vi "Test ADC Rate.vi"() -> ()   [LabVIEW 2020, in "CTI-Visa-Scratchpad.lvlib"]
uses:
  CTI-Visa-Scratchpad.lvlib
  CTI-Visa/CTI-Visa.lvlib
  <vilib>/ptbypt/NI_PtbyPt.lvlib
panel:
  in  "stop":bool
  out "ADC":dbl[][](graph)=[[2063.0, 0.0007534999895142391, 756.5504025676244]]
  in  "Port":refnum<visa-resource-name>="COM3"
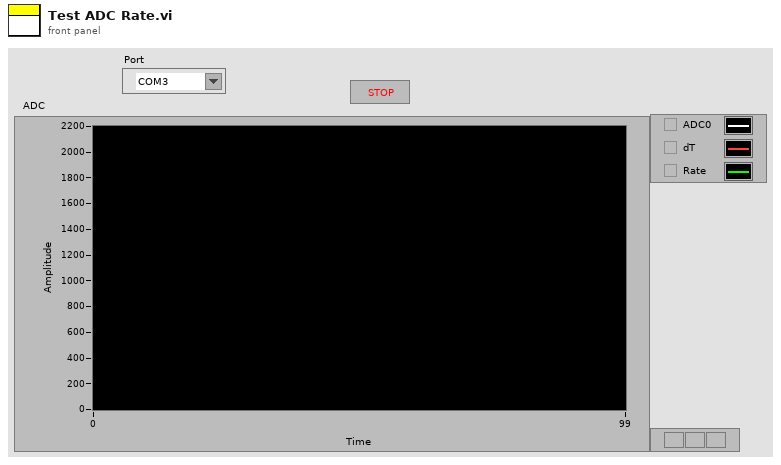
[diagram p1: front panel]
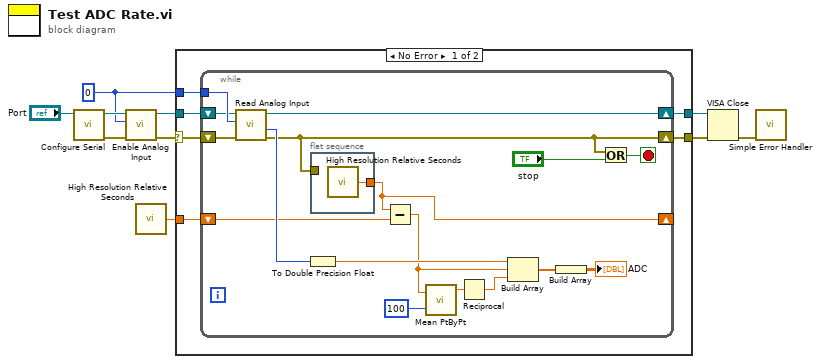
[diagram p0: block diagram]
diagram:
  w3 = 0 ("Channel")
  n1 = call "Configure Serial.vi"("VISA resource name in"="Port") -> ("error out"=w8:errorcluster, "VISA resource name"=w9:refnum<visa-resource-name>)  [unwired: 9 in]
  n2 = call "Enable Analog Input.vi"("error in (no error)"=w8, "Channel"=w3, "VISA resource name in"=w9) -> ("error out"=w7:errorcluster, "VISA resource name"=w1:refnum<visa-resource-name>)  [unwired: 7 in]
  n3 = call <vilib>:"High Resolution Relative Seconds.vi"() -> ("relative seconds"=w2:dbl)
  n4 = case shown="No Error" w7 {
    selector: w7 -> [w14 w36]
    tunnel: w1 -> [w15 w35]
    tunnel: w3 -> [w16 _]
    tunnel: [w12 w36] -> w5
    tunnel: [w13 w35] -> w6
    tunnel: w2 -> [w11 _]
    frame No Error {
      n5 = while {
        tunnel: w16 -> [w33]
        shift-right: [w30] -> w13
        shift-left: w15 -> [w32]
        shift-right: [w26] -> w12
        shift-left: w14 -> [w31]
        shift-right: [w23] -> _
        shift-left: w11 -> [w24]
        stop <- w29 stop-if-true
        n6 = call "Read Analog Input.vi"("error in (no error)"=w31, "Channel"=w33, "VISA resource name in"=w32) -> ("error out"=w26:errorcluster, "Value"=w28:u16, "VISA resource name"=w30:refnum<visa-resource-name>)  [unwired: 6 in]
        n7 = To Double Precision Float(number=w28) -> (double precision float=w22:dbl)
        n8 = flat-sequence {
          tunnel: w26 -> [_]
          tunnel: [w34] -> w23
          frame #0 {
            n9 = call <vilib>:"High Resolution Relative Seconds.vi"() -> ("relative seconds"=w34:dbl)
          }
        }
        n10 = Subtract(x=w23, y=w24) -> (x-y=w21:dbl)
        n11 = call <vilib>:"Mean PtByPt.vi"("x"=w21, "sample length"=100) -> ("mean"=w19:dbl)  [unwired: 2 in, 1 out]
        n12 = Reciprocal(x=w19) -> (1/x=w18:dbl)
        n13 = Build Array(w22, w21, w18) -> (w27:dbl[])
        n14 = Build Array(w27) -> (→"ADC":dbl[][])
        n15 = Or(x=w26, y="stop") -> (x .or. y?=w29:bool)
      }
    }
    frame Error {
    }
  }
  n16 = VISA Close(VISA resource name=w6, error in (no error)=w5) -> (error out=w4:errorcluster)
  n17 = call <vilib>:"Simple Error Handler.vi"("error in (no error)"=w4) -> ()  [unwired: 4 in, 5 out]
